vi "Save File Add Summary Data.vi"(0 "Data That Has Been\nCollecting":path, 1 "Final Weight (lbs)":string, 5 "Error In":errorcluster, 7 "Data":dbl[](array[numeric]), 8 "Use 2D String Summary":bool, 9 "Standby Power Spreadsheet":string[][](array[string]), 10 "Add Final RMC":bool, 11 "2D String Summary":string[][](array[string]), 13 "Header":string[](array[string])) -> (19 "Error Out":errorcluster)   [LabVIEW 2018]
uses:
  <vilib>/Utility/file.llb/Read Delimited Spreadsheet (string).vi
  <vilib>/Utility/file.llb/Write Delimited Spreadsheet (string).vi
panel:
  out "Summary Data":string[][](array[string])
  in  "Debug":string[][](array[string])=[["Voltage (Volts) - Mean", "Voltage (Volts) - Standard Deviation", "Voltage (Volts) - Variance", "Voltage (Volts) - Max", "Voltage (Volts) - Min", "Current (Amps) - Mean", "Current (Amps) - Standard Deviation", "Current (Amps) - Variance", "Current (Amps) - Max", "Current (Amps) - Min", "Power (Watts) - Mean", "Power (Watts) - Standard Deviation", "Power (Watts) - Variance", "Power (Watts) - Max", "Power (Watts) - Min", "WattHours - Max", "WattHours - Min", "TC Tree (AVG) - Mean", "TC Tree (AVG) - Standard Deviation", "TC Tree (AVG) - Variance", "TC Tree (AVG) - Max", "TC Tree (AVG) - Min", "Flow Rate (GPM) - Mean", "Flow Rate (GPM) - Standard Deviation", "Flow Rate (GPM) - Variance", "Flow Rate (GPM) - Max", "Flow Rate (GPM) - Min", "Gallons (Gal) - Max", "Gallons (Gal) - Min", "RTD Out (°F) - Mean", "RTD Out (°F) - Standard Deviation", "RTD Out (°F) - Variance", "RTD Out (°F) - Max", "RTD Out (°F) - Min", "RTD In (°F) - Mean", "RTD In (°F) - Standard Deviation", "RTD In (°F) - Variance", "RTD In (°F) - Max", "RTD In (°F) - Min", "RTD Ambinet (°F) - Mean", "RTD Ambient (°F) - Standard Deviation", "RTD Ambinent (°F) - Variance", "RTD Ambinent (°F) - Max", "RTD Ambinent (°F) - Min", "TC Down (°F) - Mean", "TC Down (°F) - Standard Deviation", "TC Down (°F) - Variance", "TC Down (°F) - Max", "TC Down (°F) - Min", "TC1 (°F) - Mean", "TC1 (°F) - Standard Deviation", "TC1 (°F) - Variance", "TC1 (°F) - Max", "TC1 (°F) - Min", "TC2 (°F) - Mean", "TC2 (°F) - Standard Deviation", "TC2 (°F) - Variance", "TC2 (°F) - Max", "TC2 (°F) - Min", "TC3 (°F) - Mean", "TC3 (°F) - Standard Deviation", "TC3 (°F) - Variance", "TC3 (°F) - Max", "TC3 (°F) - Min", "TC4 (°F) - Mean", "TC4 (°F) - Standard Deviation", "TC4 (°F) - Variance", "TC4 (°F) - Max", "TC4 (°F) - Min", "TC5 (°F) - Mean", "TC5 (°F) - Standard Deviation", "TC5 (°F) - Variance", "TC5 (°F) - Max", "TC5 (°F) - Min", "TC6 (°F) - Mean", "TC6 (°F) - Standard Deviation", "TC6 (°F) - Variance", "TC6 (°F) - Max", "TC6 (°F) - Min", "Total Harmonic Distortion (%V) - Max", "Total Harmonic Distortion (%V) - Min", "Frequency (Hz) - Mean ", "Frequency (Hz) - Standard Deviation", "Frequency (Hz) - Variance", "Frequency (Hz) - Max", "Frequency (Hz) - Min", "Apparent Power (VA) - Mean", "Apparent Power (VA) - Standard Deviation", "Apparent Power (VA) - Variance", "Apparent Power (VA) - Max", "Apparent Power (VA) - Min", "Power Factor - Max", "Power Factor - Min", "Current Crest Factor - Max", "Current Crest Factor - Min", "Voltage Crest Factor - Max", "Voltage Crest Factor - Min", "Elapsed Time (Sec) - Max", "Elapsed Time (Sec) - Min", "Condition Value #1", "Draw Count", ""], ["235.369", "0.114", "0.013", "235.590", "234.890", "0.142", "0.013", "0.000", "0.178", "0.136", "32.041", "1.916", "3.671", "37.360", "31.180", "1723.000", "1721.400", "128.913", "3.897", "15.188", "135.467", "120.517", "2.995", "0.085", "0.007", "3.220", "2.790", "9.460", "0.790", "110.145", "27.755", "770.359", "135.000", "71.400", "58.148", "0.559", "0.313", "60.500", "57.000", "64.519", "0.105", "0.011", "64.800", "64.300", "58.089", "0.742", "0.550", "60.300", "56.200", "135.816", "0.267", "0.071", "136.100", "134.300", "135.775", "0.247", "0.061", "136.100", "135.200", "135.590", "0.322", "0.104", "136.200", "135.000", "135.367", "0.387", "0.150", "136.000", "134.700", "129.449", "9.438", "89.082", "135.700", "100.600", "101.484", "14.884", "221.527", "134.500", "82.100", "2.252", "2.052", "59.978", "0.009", "0.000", "60.005", "59.950", "33.335", "2.998", "8.987", "41.800", "32.010", "0.975", "0.892", "4.191", "2.339", "1.402", "1.399", "188.907", "15.011", "0.000", "0.000", ""], ["234.858", "0.107", "0.012", "235.280", "234.600", "1.402", "0.047", "0.002", "1.518", "1.349", "309.376", "11.708", "137.078", "338.000", "297.600", "1761.100", "1744.000", "112.621", "4.550", "20.707", "119.917", "104.733", "3.003", "0.059", "0.003", "3.210", "2.830", "10.750", "0.790", "134.136", "0.324", "0.105", "134.500", "133.500", "57.789", "0.635", "0.403", "58.900", "56.300", "61.174", "0.490", "0.240", "62.000", "60.300", "58.032", "0.923", "0.852", "60.000", "54.900", "134.630", "0.509", "0.259", "135.300", "133.600", "134.090", "0.586", "0.343", "135.000", "132.900", "133.634", "0.699", "0.489", "134.700", "132.200", "119.908", "15.339", "235.289", "134.300", "90.300", "78.499", "8.191", "67.099", "98.200", "69.800", "74.966", "3.547", "12.580", "82.000", "69.600", "2.227", "2.033", "59.985", "0.010", "0.000", "60.012", "59.955", "329.229", "10.991", "120.810", "356.200", "317.300", "0.951", "0.932", "1.722", "1.507", "1.402", "1.398", "214.089", "15.415", "10.720", "0.000", ""], ["234.156", "0.080", "0.006", "234.380", "233.940", "1.508", "0.069", "0.005", "1.629", "1.400", "333.470", "17.040", "290.362", "363.000", "307.700", "2115.800", "2097.300", "106.906", "4.794", "22.978", "114.900", "100.333", "3.002", "0.053", "0.003", "3.150", "2.850", "10.760", "0.780", "130.824", "0.489", "0.239", "131.200", "129.600", "57.781", "0.456", "0.208", "58.600", "56.200", "57.513", "0.191", "0.036", "57.900", "57.100", "57.932", "0.697", "0.486", "59.700", "55.600", "130.771", "1.282", "1.645", "132.100", "128.200", "128.584", "2.535", "6.429", "132.000", "123.200", "111.592", "8.002", "64.029", "128.300", "104.900", "103.873", "0.944", "0.891", "104.800", "101.600", "87.744", "11.924", "142.178", "102.000", "72.400", "78.875", "5.204", "27.079", "90.400", "71.600", "3.282", "3.107", "59.987", "0.008", "0.000", "60.007", "59.966", "353.157", "16.199", "262.400", "381.500", "327.700", "0.953", "0.933", "1.701", "1.481", "1.399", "1.394", "214.804", "15.105", "10.720", "0.000", ""], ["230.639", "2.047", "4.191", "233.590", "228.430", "11.436", "7.486", "56.036", "17.316", "1.552", "2615.042", "1719.422", "2956411.942", "3968.000", "344.900", "2585.200", "2439.500", "102.561", "3.794", "14.395", "108.883", "96.817", "3.000", "0.072", "0.005", "3.200", "2.830", "10.760", "0.810", "123.074", "2.789", "7.779", "125.700", "116.300", "57.942", "0.333", "0.111", "58.800", "57.100", "57.405", "0.315", "0.099", "58.600", "56.900", "58.052", "0.751", "0.564", "60.300", "56.300", "119.712", "5.042", "25.420", "126.400", "110.700", "109.077", "3.477", "12.091", "117.600", "106.500", "106.391", "0.104", "0.011", "106.500", "106.200", "105.508", "0.473", "0.224", "105.900", "104.300", "94.515", "9.122", "83.213", "104.600", "79.600", "80.165", "5.467", "29.892", "92.600", "72.800", "3.188", "2.947", "60.015", "0.008", "0.000", "60.032", "59.994", "2622.390", "1711.612", "2929614.986", "3969.000", "361.900", "1.000", "0.950", "1.629", "1.406", "1.399", "1.394", "214.225", "15.284", "10.720", "0.000", ""], ["233.479", "0.212", "0.045", "233.830", "232.930", "0.377", "0.525", "0.276", "1.615", "0.137", "83.734", "116.142", "13488.934", "358.400", "30.870", "6070.700", "6065.800", "124.955", "5.489", "30.132", "132.617", "115.283", "3.004", "0.056", "0.003", "3.130", "2.790", "10.750", "0.790", "135.412", "0.115", "0.013", "135.500", "135.000", "57.907", "0.506", "0.256", "59.100", "56.600", "64.014", "0.208", "0.043", "64.300", "63.600", "57.903", "0.671", "0.450", "59.700", "56.300", "136.173", "0.221", "0.049", "136.400", "135.700", "135.981", "0.369", "0.136", "136.400", "135.200", "135.802", "0.403", "0.162", "136.400", "135.000", "135.536", "0.418", "0.175", "136.200", "134.700", "118.251", "23.129", "534.952", "136.000", "76.100", "87.985", "10.124", "102.502", "114.600", "75.000", "3.266", "3.022", "59.985", "0.008", "0.000", "60.009", "59.964", "87.935", "122.424", "14987.735", "376.300", "31.930", "0.968", "0.902", "3.535", "1.492", "1.400", "1.396", "214.138", "15.445", "10.720", "0.000", ""], ["233.210", "0.080", "0.006", "233.460", "232.920", "1.572", "0.095", "0.009", "1.734", "1.419", "349.608", "22.808", "520.196", "388.100", "313.700", "6426.600", "6407.200", "117.483", "4.930", "24.309", "125.300", "109.567", "3.000", "0.060", "0.004", "3.170", "2.830", "10.770", "0.790", "133.355", "0.175", "0.031", "133.600", "132.900", "57.803", "0.482", "0.233", "59.200", "56.800", "58.019", "0.238", "0.057", "58.400", "57.500", "57.988", "0.757", "0.573", "60.200", "55.700", "133.959", "0.501", "0.251", "134.400", "132.700", "133.350", "0.863", "0.745", "134.400", "131.700", "132.395", "1.510", "2.280", "134.300", "128.500", "122.888", "4.482", "20.092", "131.700", "115.700", "98.911", "15.831", "250.614", "118.000", "75.200", "83.393", "7.125", "50.771", "99.300", "73.600", "2.165", "1.935", "59.996", "0.013", "0.000", "60.032", "59.956", "366.675", "22.214", "493.462", "404.400", "331.200", "0.961", "0.943", "1.709", "1.507", "1.404", "1.399", "214.444", "15.249", "10.720", "0.000", ""]]
  # "OR"
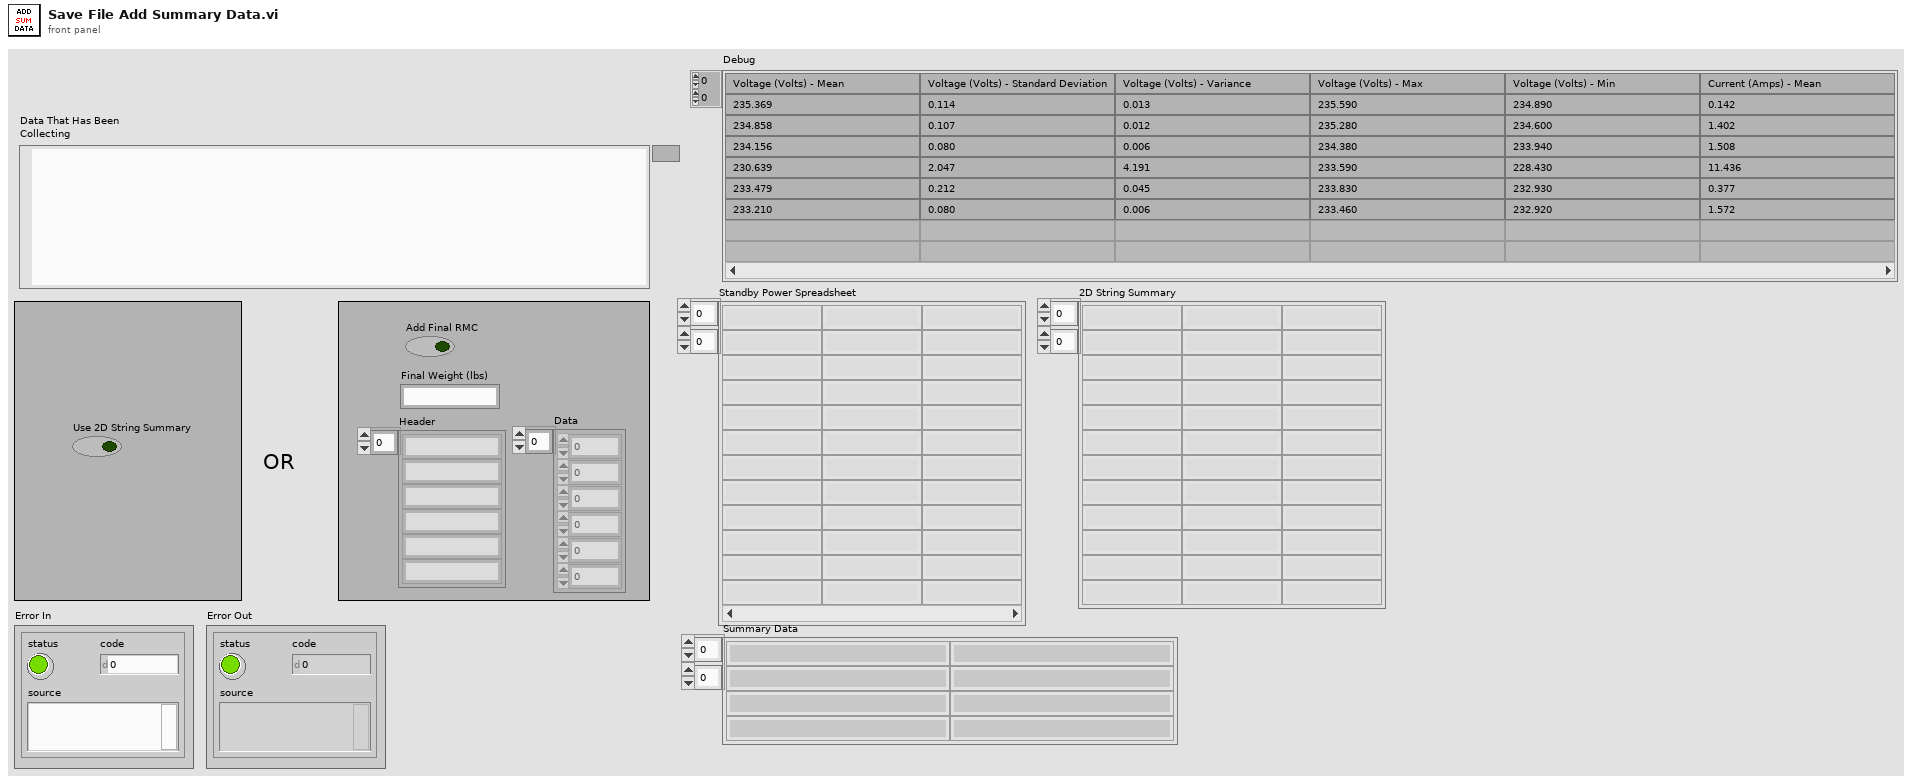
[diagram p1: front panel]
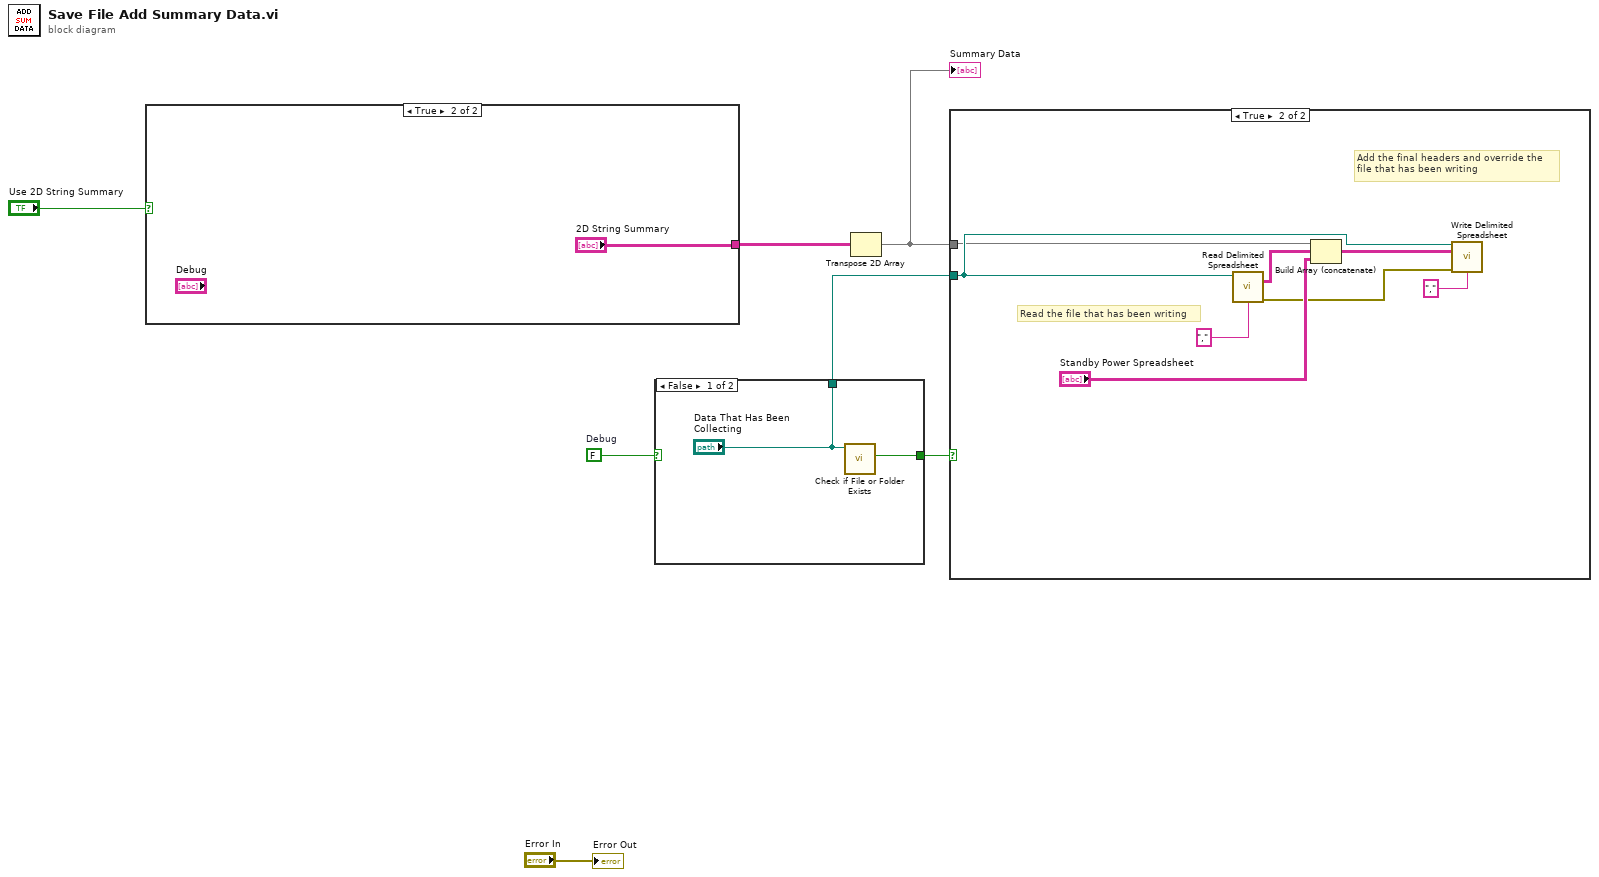
[diagram p0: block diagram]
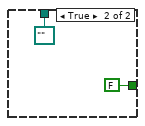
[diagram p2: hidden frame]
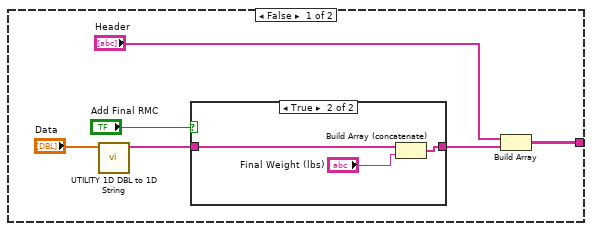
[diagram p4: hidden frame]
diagram:
  w1 = FALSE  # Debug
  n1 = case shown="True" "Use 2D String Summary" {
    tunnel: [w10 "2D String Summary"] -> w4
    frame False {
      n2 = call "UTILITY 1D DBL to 1D String.vi"("1D DBL"="Data") -> ("1D String"=w12:string[])  [unwired: 10 in]
      n3 = case shown="True" "Add Final RMC" {
        tunnel: w12 -> [w14 w17]
        tunnel: [w14 w16] -> w11
        frame False {
        }
        frame True {
          n4 = Build Array (concatenate)(w17, "Final Weight (lbs)") -> (w16:string[])
        }
      }
      n5 = Build Array("Header", w11) -> (w10:string[][])
    }
    frame True {
    }
  }
  n6 = case shown="False" w1 {
    tunnel: ["Data That Has Been\nCollecting" path "" ("Data That Has Been\nCollecting")] -> w5
    tunnel: [w19 FALSE ("file or folder exists?")] -> w2
    frame False {
      n7 = call <vilib>:"Check if File or Folder Exists.vi"("path"="Data That Has Been\nCollecting") -> ("file or folder exists?"=w19:bool)  [unwired: 8 in, 2 out]
    }
    frame True {
    }
  }
  n8 = Transpose 2D Array(2D array=w4) -> (transposed array=w3:string[][])
  "Summary Data" <- w3
  n9 = case shown="True" w2 {
    tunnel: w3 -> [_ w26]
    tunnel: w5 -> [_ w27]
    frame False {
    }
    frame True {
      # "Read the file that has been writing"
      # "Add the final headers and override the\nfile that has been writing"
      n10 = call-poly <vilib>:"Read Delimited Spreadsheet.vi"("file path (dialog if empty)"=w27, "delimiter (\\t)"="," ("delimiter (\\t)")) -> ("all rows"=w25:string[][], "error out"=w23:errorcluster)  [unwired: 8 in, 4 out]
      n11 = Build Array (concatenate)(w26, w25, "Standby Power Spreadsheet") -> (w24:string[][])
      n12 = call-poly <vilib>:"Write Delimited Spreadsheet.vi"("file path (dialog if empty)"=w27, "2D data"=w24, "error in (no error)"=w23, "delimiter (\\t)"="," ("delimiter (\\t)")) -> ()  [unwired: 10 in, 2 out]
    }
  }
  "Error Out" <- "Error In"
